vi "array -- find index.vi"(8 "number":i32, 11 "temperatures":i32[](array[numeric])=[10, 20, 56, 92, 120, 183, 194, 310]) -> (1 "left index":i32, 2 "element index":i32, 3 "element found":bool)   [LabVIEW 2010]
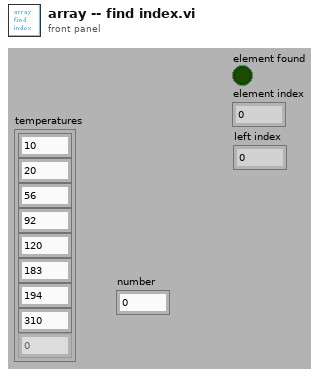
[diagram p1: front panel]
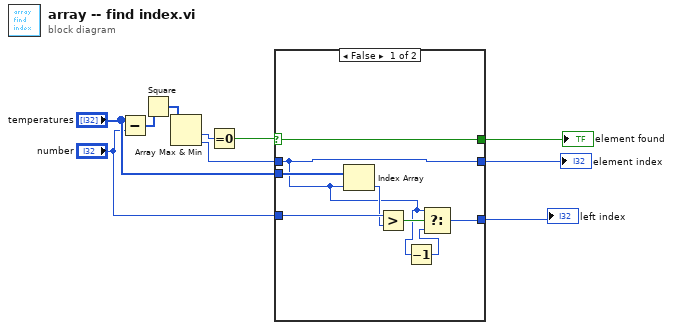
[diagram p0: block diagram]
diagram:
  n1 = Subtract(x="temperatures", y="number") -> (x-y=w9:i32[])
  n2 = Square(x=w9) -> (x^2=w8:i32[])
  n3 = Array Max & Min(array=w8) -> (min value=w10:i32, min index (indices)=w4:i32)  [unwired: 2 out]
  n4 = Equal To 0?(x=w10) -> (x = 0?=w7:bool)
  n5 = case shown="False" w7 {
    selector: w7 -> [w13 w20]
    tunnel: [w13 w20] -> w6
    tunnel: [w11 w19] -> w5
    tunnel: w4 -> [w11 w19]
    tunnel: "temperatures" -> [w18 _]
    tunnel: "number" -> [w17 _]
    tunnel: [w14 w19] -> w1
    frame False {
      n6 = Index Array(array=w18, index=w11) -> (element=w16:i32)
      n7 = Greater?(x=w17, y=w16) -> (0:w15:bool)
      n8 = Decrement(x=w11) -> (x-1=w12:i32)
      n9 = Select(t=w11, s=w15, f=w12) -> (s? t:f=w14:i32)
    }
    frame True {
    }
  }
  "element found" <- w6
  "element index" <- w5
  "left index" <- w1
